vi "Main.vi"() -> ()   [LabVIEW 2014]
doc: "This example displays an SVG image and lets you change its magnification, to demonstrate the smoothness of vector graphics at different zoom levels. It also showcases a user-defined scroll area, which is useful for containing a scene that is too large to fit on the screen (e.g. an SVG image that's magnified 20x).\n\nCopyright (c) 2019 Sze Howe Koh.\nThis code is licensed under the MIT license."
uses:
  <vilib>/addons/LQ/Qt Widgets/LQWidgetEngine/LQWidgetEngine.lvclass
  <vilib>/addons/LQ/LQ Core/Qt/Orientation.ctl
  <vilib>/addons/LQ/LQ Core/Qt/AlignmentFlag.ctl
  <vilib>/addons/LQ/LQ Core/QSize.ctl
  <vilib>/addons/LQ/Qt Widgets/QBoxLayout/Direction.ctl
  <vilib>/addons/LQ/Qwt/QwtAbstractScale/setUpperBound.vi
  <vilib>/addons/LQ/Qwt/QwtAbstractScale/setScaleStepSize.vi
  <vilib>/addons/LQ/Qwt/QwtAbstractSlider/setValue.vi
  <vilib>/addons/LQ/LQ Core/LQCoreEngine/_Polymorphic Instances/Connect_EventRefOut_DBL.vi
  <vilib>/addons/LQ/Qt GUI/LQGuiEngine/setWindowIcon.vi
  <vilib>/addons/LQ/Qt Widgets/QScrollArea/setAlignment.vi
  <vilib>/addons/LQ/Qt Widgets/QWidget/resize.vi
  <vilib>/addons/LQ/Qt Widgets/QWidget/setVisible.vi
  <vilib>/addons/LQ/Qt Widgets/QWidget/sizeHint.vi
  <vilib>/addons/LQ/LQ Core/LQCoreEngine/LQCoreEngine.lvclass
  <vilib>/addons/LQ/Qt Widgets/QBoxLayout/QBoxLayout.lvclass
  <vilib>/addons/LQ/Qwt/QwtSlider/QwtSlider.lvclass
  <vilib>/addons/LQ/LQ Core/Qt/Qt.lvlib
  <vilib>/addons/LQ/Qt SVG/QSvgWidget/QSvgWidget.lvclass
  <vilib>/addons/LQ/Qt GUI/QIcon/QIcon.lvclass
  <vilib>/addons/LQ/Qt Widgets/QScrollArea/QScrollArea.lvclass
  <vilib>/addons/LQ/Qt Widgets/QWidget/QWidget.lvclass
panel:
  in  "Stop Button":bool
  # "Prerequisite knowledge/experience\n- Basic LabVIEW programming\n- Example 3b. Connecting a Signal to a LabVIEW Event from the \"Hello World - Introduction to Widgets\"\n   series\n\n\nDescription\nThis example displays an SVG image and lets you change its magnification, to demonstrate the\nsmoothness of vector graphics at different zoom levels. It also showcases a user-defined scroll area,\nwhich is useful for containing a scene that is too large to fit on the screen (e.g. an SVG image that's\nmagnified 20x).\n\n\nShowcase\n- SVG rendering\n- User-defined scroll area"
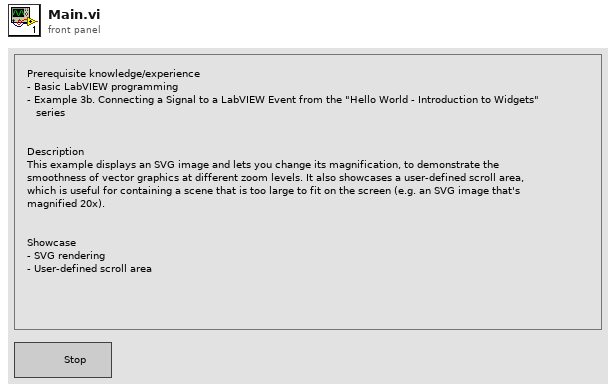
[diagram p1: front panel]
types:
  T1 = typedef "QBoxLayout.lvclass/Direction.ctl" = i32
  T2 = typedef "QSize.ctl" = cluster{"width":i32, "height":i32}
  T3 = typedef "Qt.lvlib/AlignmentFlag.ctl" = i32
  T4 = typedef "Qt.lvlib/Orientation.ctl" = i32
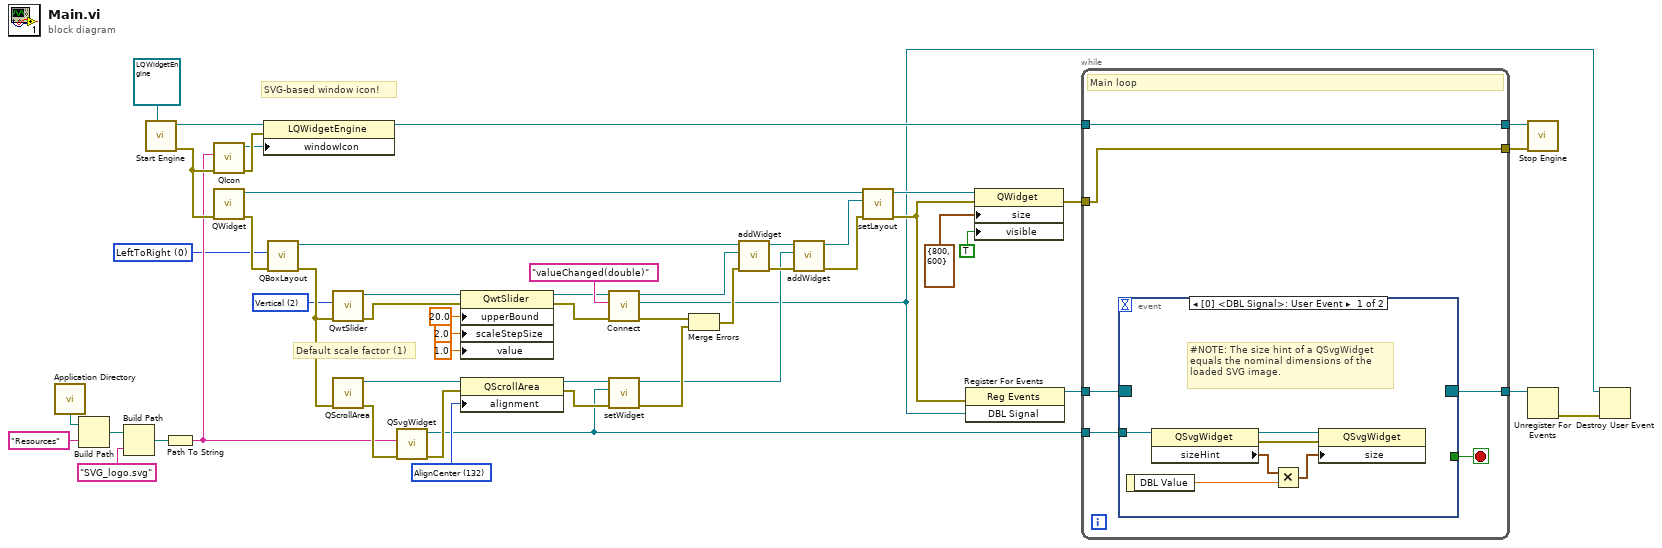
[diagram p0: block diagram]
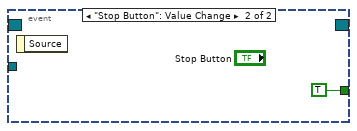
[diagram p2: hidden frame]
diagram:
  w7 = T1 0 items=["LeftToRight", "RightToLeft", "TopToBottom", "BottomToTop"] ("direction")
  w32 = T3 132 items=["AlignLeading"=1, "AlignTrailing"=2, "AlignHCenter"=4, "AlignJustify"=8, "AlignAbsolute"=16, "AlignHorizontal_Mask"=31, "AlignTop"=32, "AlignBottom"=64, "AlignVCenter"=128, "AlignBaseline"=256, "AlignVertical_Mask"=480, "AlignCenter"=132] ("alignment")
  w42 = T4 2 items=["Horizontal"=1, "Vertical"=2] ("orientation")
  # "Default scale factor (1)"
  # "SVG-based window icon!"
  n1 = call <vilib>:"Application Directory.vi"() -> ("Application Directory"=w40:path)
  n2 = Build Path(base path=w40, name or relative path="Resources") -> (appended path=w38:path)
  n3 = Build Path(base path=w38, name or relative path="SVG_logo.svg" ("fileName")) -> (appended path=w37:path)
  n4 = call <vilib>:"Start Engine.vi"("Engine Type"=refnum<class "LQWidgetEngine.lvclass"> refnum ("Qt Widgets.lvlib:LQWidgetEngine")) -> ("Error Out"=w46:errorcluster, "New Engine"=w41:refnum<class "LQWidgetEngine.lvclass">)  [unwired: 9 in]
  n5 = Path To String(path=w37) -> (string=w36:string)
  n6 = call <vilib>:"QIcon.vi"("Error In"=w46, "fileName"=w36) -> ("Error Out"=w45:errorcluster, "New QIcon"=w34:refnum<class "QIcon.lvclass">)  [unwired: 8 in]
  n7 = call <vilib>:"QWidget.vi"("Error In"=w46) -> ("Error Out"=w47:errorcluster, "New QWidget"=w25:refnum<class "QWidget.lvclass">)  [unwired: 9 in]
  n8 = property class="LQWidgetEngine"(reference=w41, error in=w45, "windowIcon"=w34) -> (reference out=w20:refnum<class "LQWidgetEngine.lvclass">)  [unwired: 1 out]
  n9 = call <vilib>:"QBoxLayout.vi"("Error In"=w47, "direction"=w7) -> ("Error Out"=w48:errorcluster, "New QBoxLayout"=w29:refnum<class "QBoxLayout.lvclass">)  [unwired: 8 in]
  n10 = call <vilib>:"QwtSlider.vi"("Error In"=w48, "orientation"=w42) -> ("Error Out"=w6:errorcluster, "New QwtSlider"=w14:refnum<class "QwtSlider.lvclass">)  [unwired: 8 in]
  n11 = call <vilib>:"QScrollArea.vi"("Error In"=w48) -> ("Error Out"=w49:errorcluster, "New QScrollArea"=w33:refnum<class "QScrollArea.lvclass">)  [unwired: 9 in]
  n12 = call <vilib>:"QSvgWidget.vi"("Error In"=w49, "file"=w36) -> ("Error Out"=w44:errorcluster, "New QSvgWidget"=w19:refnum<class "QSvgWidget.lvclass">)  [unwired: 8 in]
  n13 = property class="QwtSlider"(reference=w14, error in=w6, "upperBound"=20.0, "scaleStepSize"=2.0 ("value"), "value"=1.0 ("scaleStepSize")) -> (reference out=w13:refnum<class "QwtSlider.lvclass">, error out=w5:errorcluster)
  n14 = property class="QScrollArea"(reference=w33, error in=w44, "alignment"=w32) -> (reference out=w31:refnum<class "QScrollArea.lvclass">, error out=w30:errorcluster)
  n15 = call-poly <vilib>:"Connect.vi"("Error In"=w5, "Signal Signature"="valueChanged(double)", "Sender In"=w13) -> ("Error Out"=w4:errorcluster, "DBL Signal"=w17:refnum<user-event>, "Sender Out"=w15:refnum<class "QwtSlider.lvclass">)  [unwired: 6 in]
  n16 = call <vilib>:"setWidget.vi"("Error In"=w30, "widget"=w19, "QScrollArea In"=w31) -> ("Error Out"=w50:errorcluster, "QScrollArea Out"=w27:refnum<class "QScrollArea.lvclass">)  [unwired: 7 in]
  n17 = Merge Errors(w4, w50) -> (w51:errorcluster)
  n18 = call <vilib>:"addWidget.vi"("Error In"=w51, "widget"=w15, "QBoxLayout In"=w29) -> ("Error Out"=w52:errorcluster, "QBoxLayout Out"=w28:refnum<class "QBoxLayout.lvclass">)  [unwired: 7 in]
  n19 = call <vilib>:"addWidget.vi"("Error In"=w52, "widget"=w27, "QBoxLayout In"=w28) -> ("Error Out"=w3:errorcluster, "QBoxLayout Out"=w24:refnum<class "QBoxLayout.lvclass">)  [unwired: 7 in]
  n20 = call <vilib>:"setLayout.vi"("Error In"=w3, "layout"=w24, "QWidget In"=w25) -> ("Error Out"=w53:errorcluster, "QWidget Out"=w23:refnum<class "QWidget.lvclass">)  [unwired: 7 in]
  n21 = register-events(error in=w53, w17) -> (reference out=w22:refnum<event-registration>)  [unwired: 1 in, 1 out]
  n22 = property class="QWidget"(reference=w23, error in=w53, "size"=T2 {"width"=800, "height"=600} ("minimumSize"), "visible"=TRUE) -> (error out=w2:errorcluster)  [unwired: 1 out]
  n23 = while {
    tunnel: w22 -> [w59]
    tunnel: [w58] -> w21
    tunnel: w20 -> [w58]
    tunnel: w19 -> [w56]
    tunnel: [w55] -> w18
    tunnel: w2 -> [w54]
    tunnel: [w54] -> w1
    stop <- w57 stop-if-true
    # "Main loop"
    n24 = event shown="[0] <DBL Signal>: User Event" {
      selector: w59 -> [_ _]
      dyn-events: [_ _] -> w55
      timeout: _ -> [_ _]
      tunnel: [_ TRUE] -> w57
      tunnel: w56 -> [w65 _]
      event User Event {
        # "#NOTE: The size hint of a QSvgWidget\nequals the nominal dimensions of the\nloaded SVG image."
        n25 = event-data() -> ("DBL Value"=w63:dbl)  [unwired: 1 in]
        n26 = property class="QSvgWidget"(reference=w65) -> (reference out=w64:refnum<class "QSvgWidget.lvclass">, error out=w60:errorcluster, "sizeHint"=w62:T2)  [unwired: 1 in]
        n27 = Multiply(x=w62, y=w63) -> (x*y=w61:cluster{"width":dbl, "height":dbl})
        n28 = property class="QSvgWidget"(reference=w64, error in=w60, "size"=w61) -> ()  [unwired: 2 out]
      }
      event "Stop Button": Value Change {
        n29 = event-data() -> ()  [unwired: 1 in, 1 out]
      }
    }
  }
  n30 = call <vilib>:"Stop Engine.vi"("Error In"=w1, "LQCoreEngine"=w21) -> ()  [unwired: 9 in, 1 out]
  n31 = Unregister For Events(event registration refnum=w18) -> (error out=w16:errorcluster)  [unwired: 1 in]
  n32 = Destroy User Event(user event=w17, error in=w16) -> ()  [unwired: 1 out]
